vi "Test GUI.vi"() -> ()   [LabVIEW 2018]
doc: "Acoustic Test for EOL"
uses:
  Types/EnumType.ctl
  <vilib>/Utility/miscctls.llb/LVRowAndColumnTypeDef.ctl
  <vilib>/Utility/miscctls.llb/LVRowAndColumnUnsignedTypeDef.ctl
  <vilib>/Utility/error.llb/DialogType.ctl
  Supports/Global 1.vi
panel:
  out "SN":u16
  in  "ZEBRA PRINT ME74":bool
  in  "Reset Conter 2":bool
  out "TARGET COUNTER":dbl
  in  "PLAN TARGET":dbl
  out "CounterFull 2":bool
  out "Buffer 2":u16
  out "Buffer":u16
  out "MIC 2":cluster{dbl[], dbl[]}[](graph)
  out "Test Data":string[][](table)
  out "MIC 1":cluster{dbl[], dbl[]}[](graph)
  in  "Change Model":bool
  in  "Alarm":u16
  out "Alarm Display":string
  out "MCError":bool
  out "Auto Running":bool
  out "CYCLE\nTIME":u16
  out "ME79Model":bool
  in  "Reset Conter":bool
  out "NG":dbl
  out "OK":dbl
  in  "BOX TARGET":dbl
  out "CounterFull":bool
  out "File Open Reference out":T1
  out "Test Error":bool
  out "Power OK":bool
  in  "Print":bool=TRUE
  out "LBL Data":T2
  in  "Cal Mic CH":bool
  out "AT Cond 2":bool
  out "AT Cond":bool
  in  "IAI Cal":bool
  in  "IAI Ret":bool
  in  "IAI Adv":bool
  out "Status":string
  in  "Calibrate":bool
  out "Connection":bool
  out "Stop":bool
  out "Start":bool
  out "Error":bool
  out "Fail":bool
  out "Pass":bool
  out "Done":bool
  out "Busy":bool
  out "Ready":bool
  in  "Channel":bool
  out "Model":bool
  in  "Start":bool
  in  "Mode":bool
  in  "Quit":bool
  out "Test Result":bool
  out "Test Running":bool
  # "MICROPHONE TEST EOL"
  # "TEST DATA"
  # "MANUAL CONTROL"
  # "BUFFER\nE180639"
  # "BUFFER\nE183362"
  # "Version 2.1 Build 20200305"
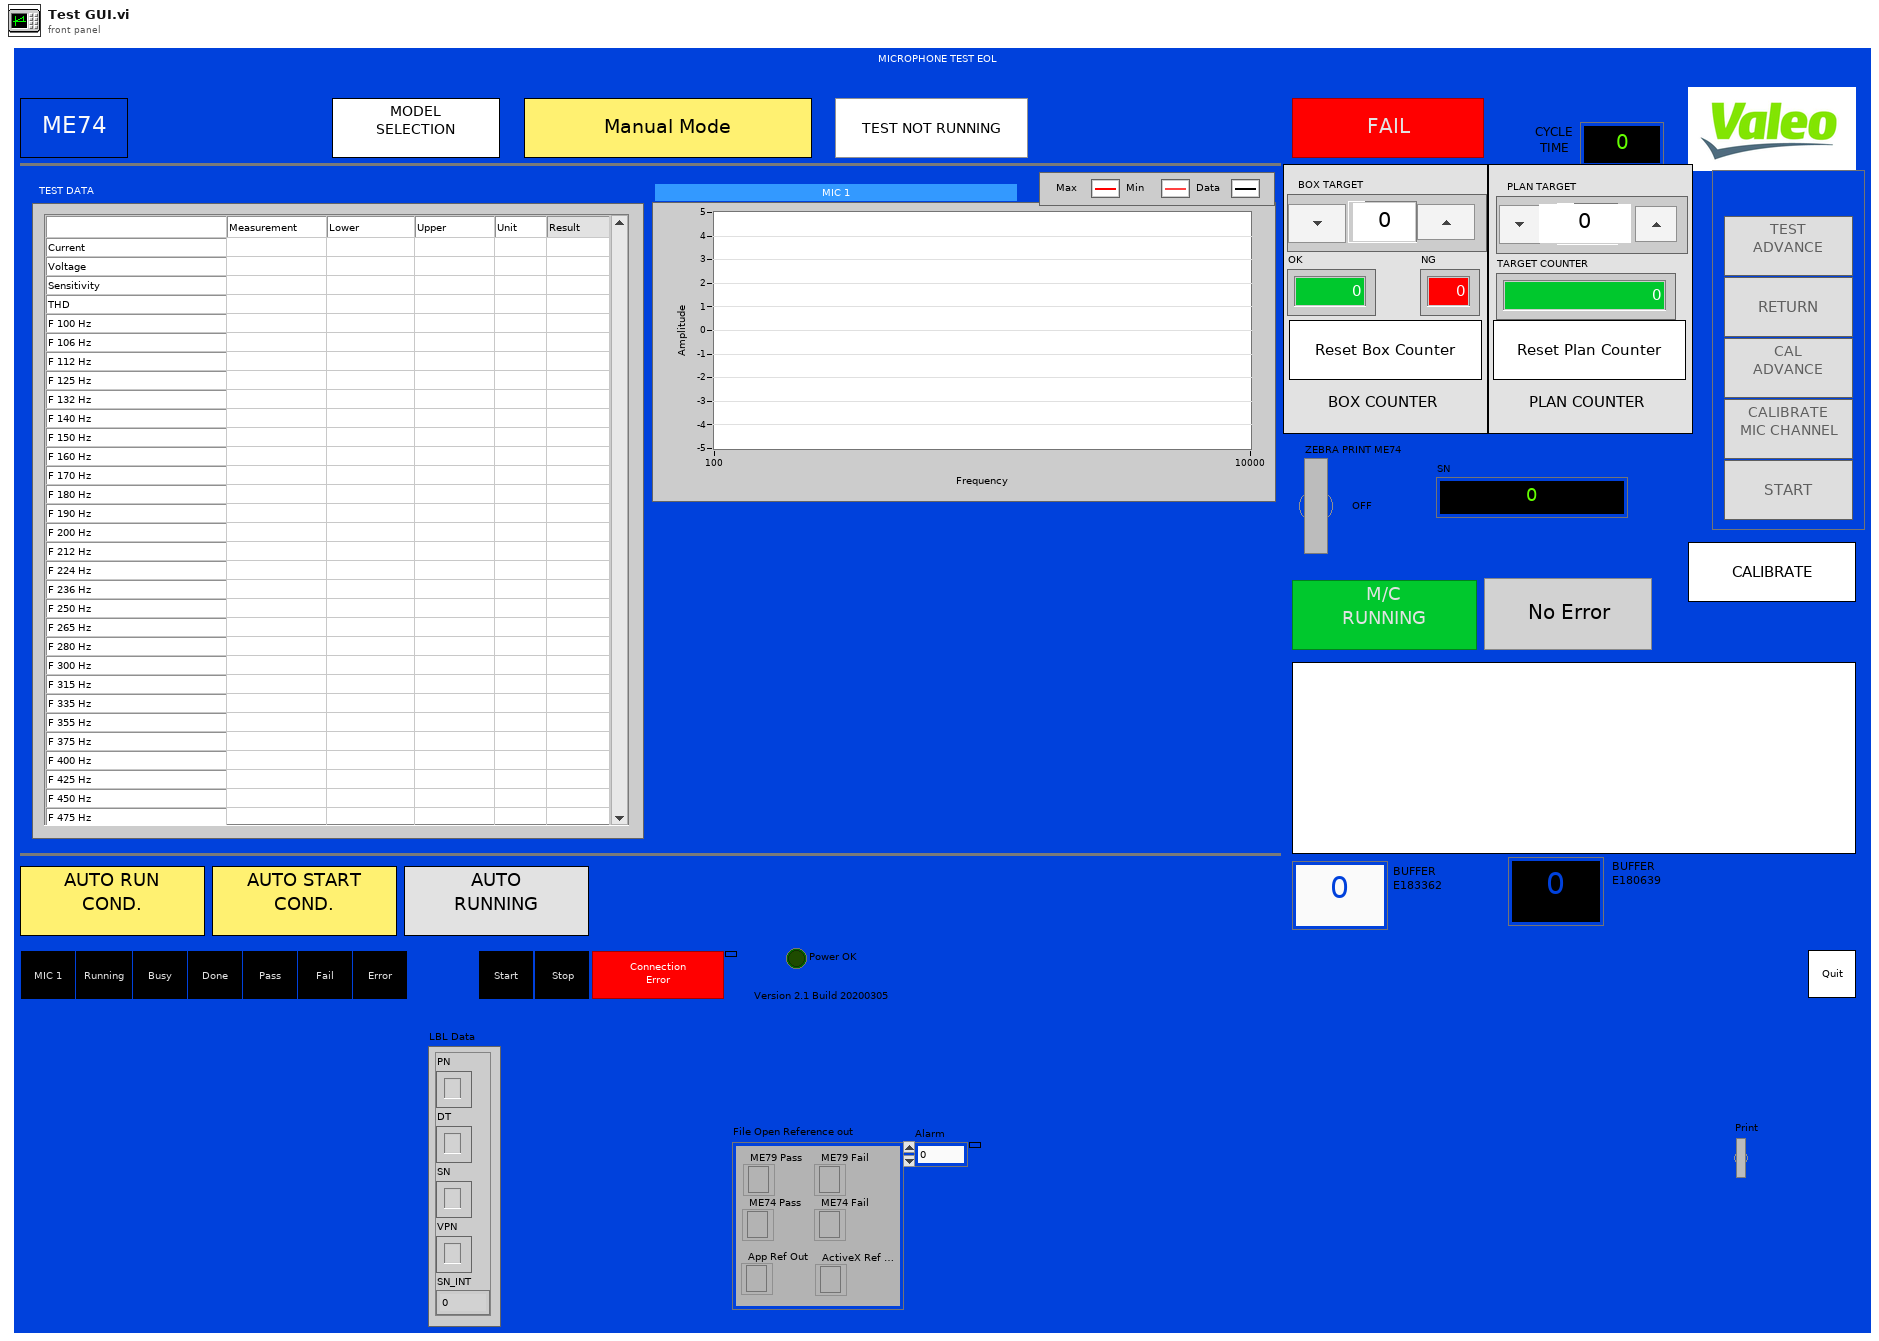
[diagram p1: front panel]
types:
  T1 = cluster{"ME79 Pass":refnum<k7>, "ME79 Fail":refnum<k7>, "ME74 Pass":refnum<k7>, "ME74 Fail":refnum<k7>, "App Ref Out":refnum<k7>, "ActiveX Ref Out":refnum<k7>}
  T2 = cluster{"PN":string, "DT":string, "SN":string, "VPN":string, "SN_INT":i32}
  T3 = typedef "EnumType.ctl" = enum16{"Initial", "Wait PLC Connect", "Ready", "Load and Init Config", "Power Supply On", "Freq Sweep 1", "Freq Sweep 2", "Power Supply Off", "Save Test Data", "Print Label", "Display Result", "Quit", "Calibration"}
  T4 = enum8{"Enabled", "Disabled", "Disabled and Grayed Out"}
  T5 = typedef "LVRowAndColumnTypeDef.ctl" = cluster{"Row":i32, "Column":i32}
  T6 = typedef "LVRowAndColumnUnsignedTypeDef.ctl" = cluster{"Row":u32, "Column":u32}
  T7 = typedef "LimitType.ctl" = cluster{"PSU":cluster{"Current Lower (mA)":dbl, "Current Upper (mA)":dbl, "Voltage Lower (V)":dbl, "Voltage Upper (V)":dbl}, "Mic":cluster{"Sensitivity (mV/Pa)":cluster{"Lower":dbl, "Upper":dbl}, "THD (%)":cluster{"Lower":dbl, "Upper":dbl}, "Freq Response":cluster{"Freq":dbl, "Upper":dbl, "Lower":dbl}[]}}
  T8 = typedef "ConfigurationType.ctl" = cluster{"PSU Setting":T9, "Sweep Settings":T10}
  T9 = typedef "SupplyConfig.ctl" = cluster{"Channel Name":string, "Source Delay (Sec)":dbl, "Measurement:Sense":i32, "voltage level":dbl, "voltage level range":dbl, "current limit":dbl, "current limit range":dbl, "resource name":refnum<k15>}
  T10 = typedef "Peiker_Stepped Sweep Settings.ctl" = cluster{"Input Settings":cluster{"IEPE min time to settle [s]":dbl, "Responce Channel Settings":cluster{"DSA response channel settings":T11, "response channel info":T12, "AI response settings":cluster{"response channel":tag, "max value [V]":dbl, "min value [V]":dbl, "terminal configuration":i32}}, "Stimulus Channel Settings":cluster{"AI stimulus settings":cluster{"stimulus channel":tag, "max value [V]":dbl, "min value [V]":dbl, "terminal configuration":i32}, "DSA stimulus channel settings":T11, "stimulus channel info":T12}}, "Output Settings":cluster{"AO source settings":cluster{"excitation channel":tag, "max value [V]":dbl, "min value [V]":dbl, "terminal configuration":i32}}}
  T11 = typedef "svc_DSA Channel Settings.ctl" = cluster{"coupling":i32, "enable IEPE excitation":bool, "IEPE current [mA]":dbl}
  T12 = typedef "svc_Channel Info.ctl" = cluster{"sensor sensitivity":dbl, "engineering units":T13, "dB reference":dbl, "custom label":string, "weighting filter":T14, "pregain":dbl}
  T13 = typedef "svc_Engineering Units Text Ring.ctl" = u16
  T14 = typedef "svc_Weighting Filter Text Ring.ctl" = u16
  T15 = cluster{"Label Data":string, "Label Data":string, "Label Data":string, "Label Data":string, "Cycle Time (ms)":i32}
  T16 = typedef "DialogType.ctl" = u16
  T17 = cluster{"frequency [Hz]":dbl[], "amplitude":dbl[]}
  T18 = cluster{string, "DT":string, "SN":string, "date/time string":string, "LINECODE":string, "NG CODE OUT":string}
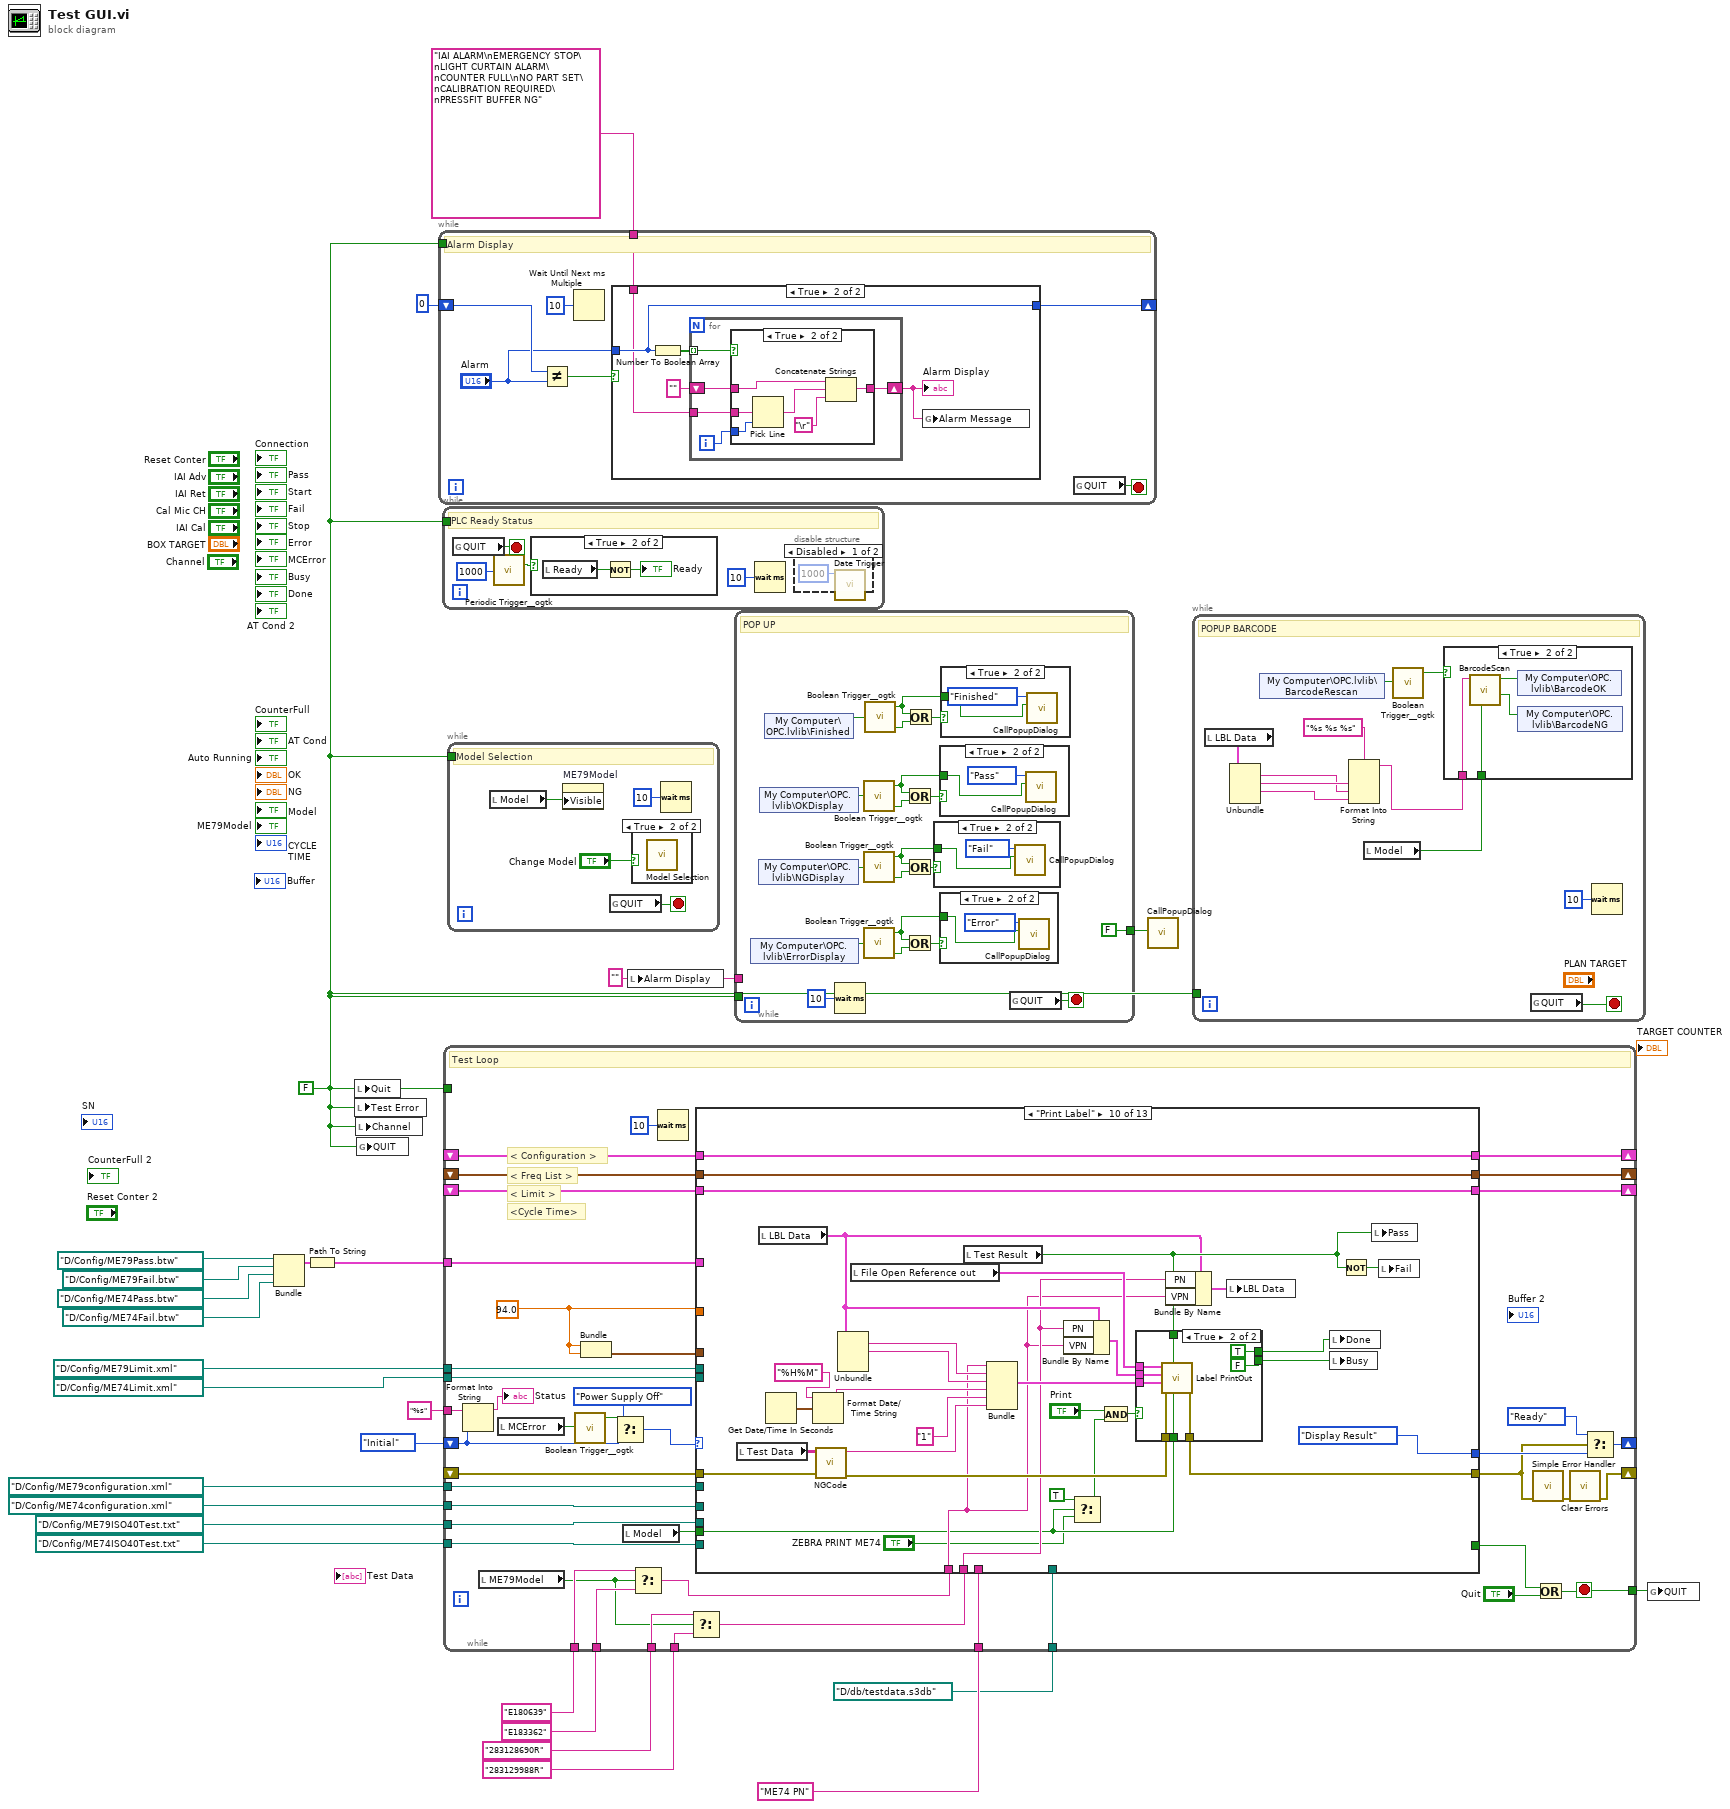
[diagram p0: block diagram]
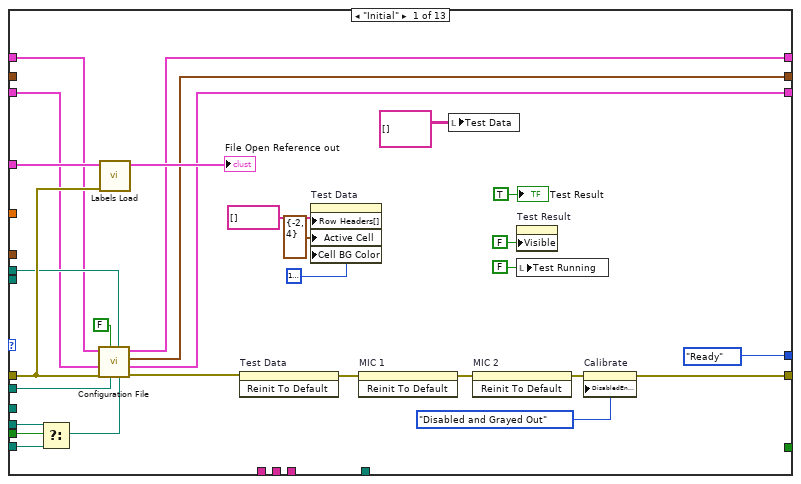
[diagram p12: hidden frame]
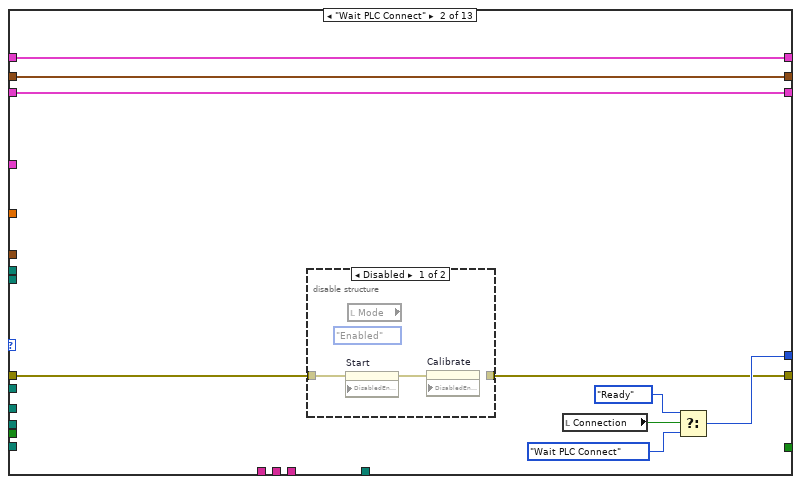
[diagram p13: hidden frame]
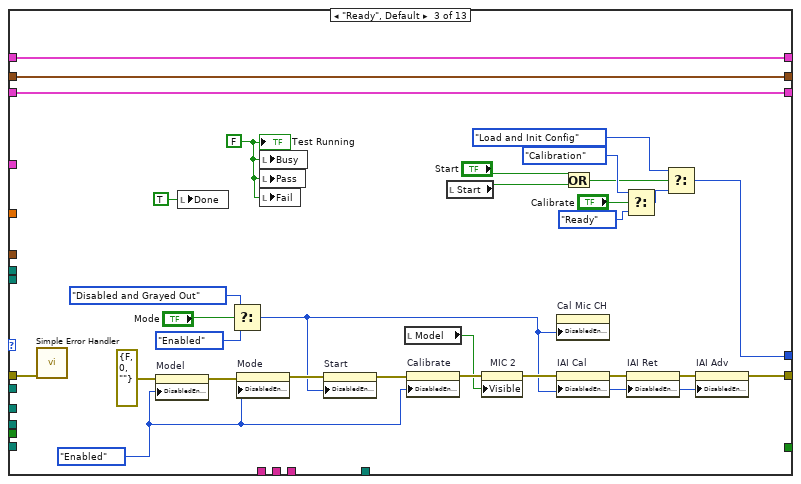
[diagram p15: hidden frame]
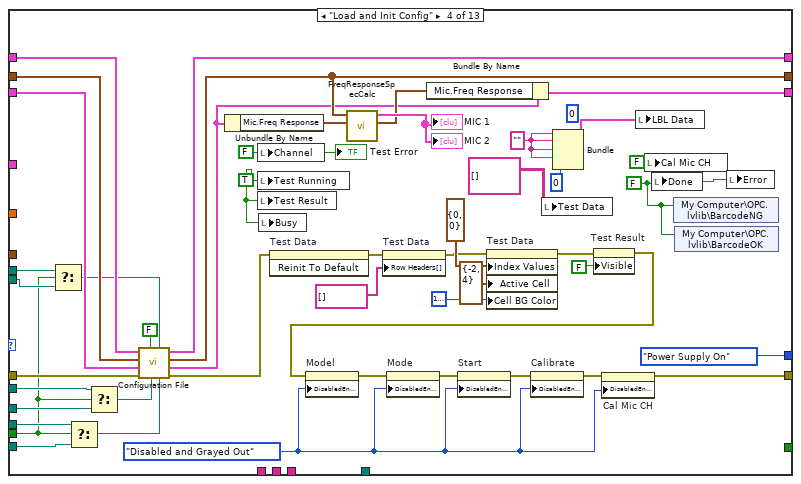
[diagram p16: hidden frame]
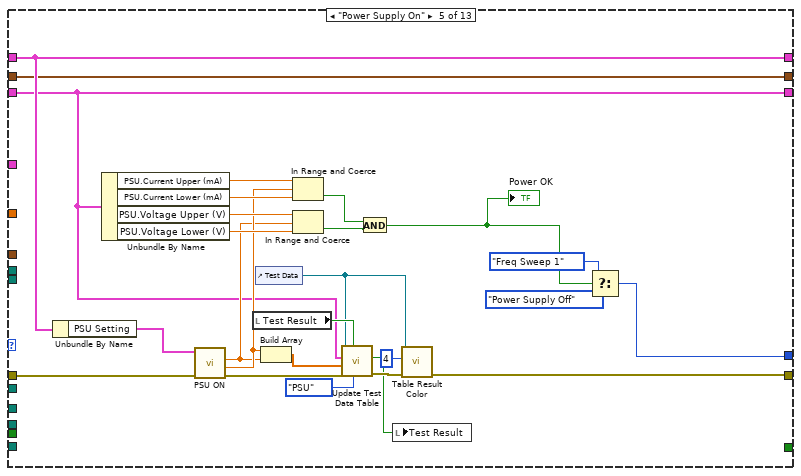
[diagram p17: hidden frame]
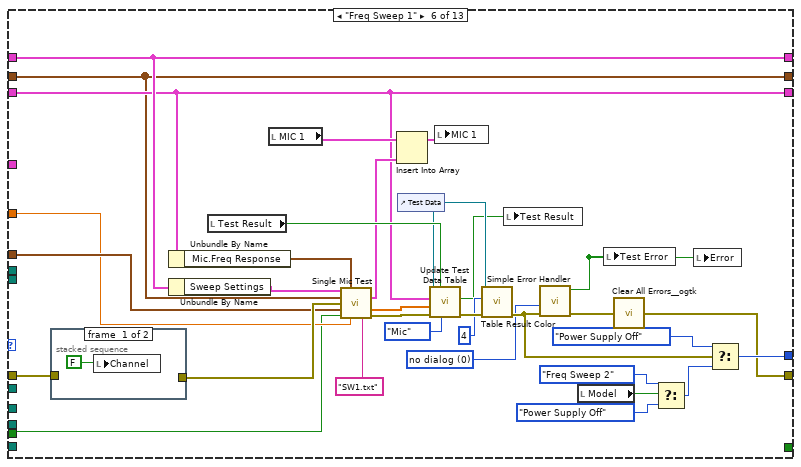
[diagram p18: hidden frame]
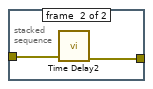
[diagram p19: hidden frame]
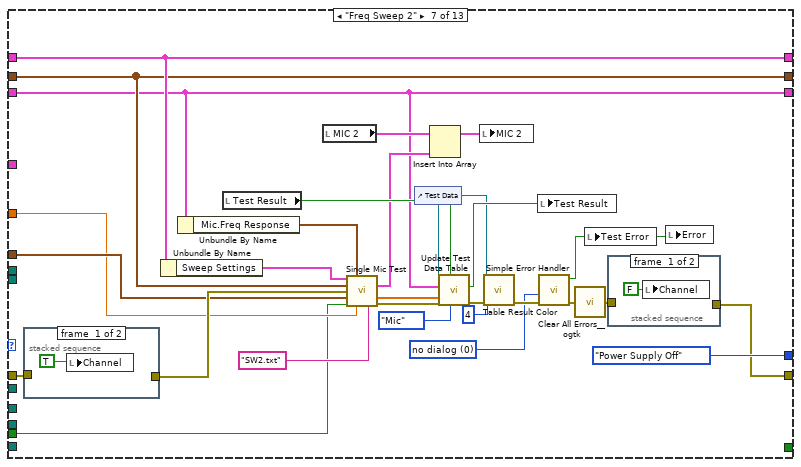
[diagram p20: hidden frame]
diagram:
  w2 = ""
  w1 = FALSE ("Quit")
  n1 = Bundle(path "D:/Config/ME79Pass.btw", path "D:/Config/ME79Fail.btw", path "D:/Config/ME74Pass.btw", path "D:/Config/ME74Fail.btw") -> (w23:cluster{path, path, path, path})  [unwired: 1 in]
  n2 = Path To String(path=w23) -> (string=w24:cluster{string, string, string, string})
  n3 = local write "Quit"(w1) -> ()
  n4 = local write "Test Error"(w1) -> ()
  n5 = local write "Channel"(w1) -> ()
  n6 = global write "Global 1.vi" "QUIT"(w1) -> ()
  n7 = while {
    shift-right: [w30] -> _
    shift-left: u16 0 -> [w32]
    tunnel: w1 -> [_]
    tunnel: "IAI ALARM\nEMERGENCY STOP\nLIGHT CURTAIN ALARM\nCOUNTER FULL\nNO PART SET\nCALIBRATION REQUIRED\nPRESSFIT BUFFER NG" -> [w28]
    stop <- w27 stop-if-true
    # "Alarm Display"
    n8 = Not Equal?(x=w32, y="Alarm") -> (x != y?=w31:bool)
    n9 = Wait Until Next ms Multiple(millisecond multiple=u32 10) -> ()  [unwired: 1 out]
    n10 = case shown="True" w31 {
      tunnel: [w34 w37] -> w30
      tunnel: "Alarm" -> [w34 w37]
      tunnel: w28 -> [_ w36]
      frame False {
      }
      frame True {
        n11 = Number To Boolean Array(number=w37) -> (Boolean array=w39:bool[])
        n12 = for {
          tunnel: w39 -> [w44] mode=indexing
          shift-right: [w41] -> w35
          shift-left: "" -> [w40]
          tunnel: w36 -> [w42]
          i -> [w43]
          n13 = case shown="True" w44 {
            tunnel: w43 -> [_ w51]
            tunnel: w42 -> [_ w50]
            tunnel: w40 -> [w45 w48]
            tunnel: [w45 w49] -> w41
            frame False {
            }
            frame True {
              n14 = Pick Line(multi-line string=w50, line index=w51) -> (output string=w47:string)  [unwired: 1 in]
              n15 = Concatenate Strings(w48, w47, "\r") -> (w49:string)
            }
          }
        }
        "Alarm Display" <- w35
        n16 = global write "Global 1.vi" "Alarm Message"(w35) -> ()
      }
    }
    n17 = global read "Global 1.vi" "QUIT"() -> (w27:bool)
  }
  n18 = while {
    tunnel: w1 -> [_]
    stop <- w52 stop-if-true
    # "PLC Ready Status"
    n19 = global read "Global 1.vi" "QUIT"() -> (w52:bool)
    n20 = call <userlib>:"Periodic Trigger__ogtk.vi"("time (ms)"=u32 1000 ("y")) -> ("Triggered"=w55:bool)  [unwired: 12 in, 2 out]
    n21 = case shown="True" w55 {
      frame False {
      }
      frame True {
        n22 = local read "Ready"() -> (w57:bool)
        n23 = Not(x=w57) -> (.not. x?=→"Ready":bool)
      }
    }
    n24 = Wait (ms)(milliseconds to wait=u32 10) -> ()  [unwired: 1 out]
    n25 = disable-structure shown="Disabled" {
      frame Disabled {
        n26 = call "Date Trigger.vi"("y"=u32 1000) -> ()  [unwired: 11 in]
      }
      frame Enabled {
      }
    }
  }
  n27 = while {
    shift-right: [w88] -> _
    shift-left: EnumType."Initial" ("Enum") -> [w71]
    shift-right: [w86] -> _
    shift-left: _ -> [w100]
    tunnel: path "D:/Config/ME79configuration.xml" -> [w99]
    shift-right: [w98] -> _
    shift-left: _ -> [w97]
    shift-right: [w95] -> _
    shift-left: _ -> [w96]
    tunnel: path "D:/Config/ME79ISO40Test.txt" -> [w94]
    shift-right: [w92] -> _
    shift-left: _ -> [w93]
    tunnel: path "D:/Config/ME79Limit.xml" -> [w91]
    tunnel: path "D:/db/testdata.s3db" -> [w85]
    tunnel: path "D:/Config/ME74ISO40Test.txt" -> [w83]
    tunnel: w1 -> [_]
    tunnel: "ME74 PN" -> [w80]
    tunnel: w24 -> [w77]
    tunnel: "E180639" -> [w75]
    tunnel: "E183362" -> [w74]
    tunnel: "283128690R" -> [w67]
    tunnel: "283129988R" -> [w66]
    tunnel: path "D:/Config/ME74configuration.xml" -> [w64]
    tunnel: path "D:/Config/ME74Limit.xml" -> [w63]
    tunnel: "%s" ("format string") -> [w60]
    tunnel: [w59] -> w3
    stop <- w59 stop-if-true
    w73 = 94.0 ("dB Reference")
    # "<Cycle Time>"
    # "< Limit >"
    # "< Freq List >"
    # "< Configuration >"
    # "Test Loop"
    n28 = Format Into String(format string=w60, w71) -> (resulting string=→"Status":string)  [unwired: 2 in, 1 out]
    n29 = local read "ME79Model"() -> (w62:bool)
    n30 = local read "MCError"() -> (w69:bool)
    n31 = call <userlib>:"Boolean Trigger__ogtk.vi"("Boolean Input"=w69) -> ("Rising Edge"=w68:bool)  [unwired: 1 in, 1 out]
    n32 = Bundle("dB Reference"=w73, "dB Reference"=w73) -> (w79:cluster{"dB Reference":dbl, "dB Reference":dbl})  [unwired: 1 in]
    n33 = Select(t=EnumType."Power Supply Off" ("Enum"), s=w68, f=w71) -> (s? t:f=w70:T3)
    n34 = local read "Model"() -> (w84:bool)
    n35 = Select(t=w75, s=w62, f=w74) -> (s? t:f=w76:string)
    n36 = Wait (ms)(milliseconds to wait=u32 10) -> ()  [unwired: 1 out]
    n37 = Select(t=w67, s=w62, f=w66) -> (s? t:f=w65:string)
    n38 = case shown="\"Print Label\"" w70 {
      tunnel: w100 -> [w115 w132 w169 w218 w245 w269 w301 w330 w361 w390 w424 w457 w464]
      tunnel: [w120 w131 w149 w186 w224 w249 w299 w332 w357 w404 w425 w457 w461] -> w78
      tunnel: [EnumType."Ready" ("Enum") w138 w164 EnumType."Power Supply On" ("Enum") w236 w252 EnumType."Power Supply Off" ("Enum") w322 EnumType."Print Label" ("Enum") EnumType."Display Result" ("Enum") EnumType."Ready" ("Enum") EnumType."Quit" ("Enum") EnumType."Ready" ("Enum")] -> w90
      tunnel: [_ _ _ _ _ _ _ _ _ _ _ TRUE _] -> w82
      tunnel: w99 -> [w113 _ _ w180 _ _ _ _ _ _ _ _ _]
      tunnel: [w106 w137 w172 w216 w229 w278 w310 w334 w364 w408 w429 w455 w472] -> w98
      tunnel: w97 -> [w105 w137 w172 w215 w229 w278 w310 w334 w364 w408 w429 w455 w472]
      tunnel: [w104 w136 w171 w193 w223 w255 w308 w336 w340 w407 w428 w454 w473] -> w95
      tunnel: w96 -> [_ w136 w171 w214 w223 w255 w308 w336 w340 w407 w428 w454 w473]
      tunnel: w94 -> [w111 _ _ w206 _ _ _ _ _ _ _ _ w469]
      tunnel: w93 -> [w102 w135 w170 w213 w222 w258 w289 w335 w363 w406 w427 w453 w474]
      tunnel: [w103 w135 w170 w209 w222 w258 w289 w335 w363 w406 w427 w453 w474] -> w92
      tunnel: w91 -> [w108 _ _ w178 _ _ _ _ _ _ _ _ _]
      tunnel: w85 -> [_ _ _ _ _ _ _ _ w360 _ _ _ w465]
      tunnel: w84 -> [w112 _ _ w176 _ w246 w282 _ w338 w382 _ _ w471]
      tunnel: w83 -> [w110 _ _ w205 _ _ _ _ _ _ _ _ w468]
      tunnel: w79 -> [_ _ _ _ _ w264 w295 _ _ _ _ _ _]
      tunnel: w73 -> [_ _ _ _ _ w263 w294 _ _ _ _ _ _]
      tunnel: w76 -> [_ _ _ _ _ _ _ _ w354 w384 _ _ _]
      tunnel: w80 -> [_ _ _ _ _ _ _ _ w353 _ _ _ _]
      tunnel: w77 -> [w117 _ _ _ _ _ _ _ _ _ _ _ _]
      tunnel: w65 -> [_ _ _ _ _ _ _ _ _ w385 _ _ _]
      tunnel: w64 -> [_ _ _ w181 _ _ _ _ _ _ _ _ _]
      tunnel: w63 -> [_ _ _ w177 _ _ _ _ _ _ _ _ _]
      frame "Initial" {
        n39 = Select(t=w111, s=w112, f=w110) -> (s? t:f=w109:path)
        n40 = call "Configuration File.vi"("Freq List File"=w109, "Limit File"=w108, "Configurtion File"=w113, "Mode (F-Read)"=FALSE, "Error In"=w115, "Limit"=w102, "Configuration"=w105) -> ("Error Out"=w114:errorcluster, "Limit Out"=w103:T7, "Freq List Out"=w104:cluster{"Freq":dbl, "Amp":dbl}[], "value"=w106:T8)  [unwired: 1 in]
        n41 = call "Labels Load.vi"("error in (no error)"=w115, "Labels"=w117) -> ("File Open Reference out"=→"File Open Reference out":T1)  [unwired: 8 in, 1 out]
        n42 = invoke on="Test Data" class="Tbl (strict)" method="Reinit To Default"(error in=w114) -> (error out=w128:errorcluster)  [unwired: 2 in, 2 out]
        n43 = property on="Test Data" class="Tbl (strict)"("Row Headers[]"=string[] [], "Active Cell"=T5 {"Row"=-2, "Column"=4} ("Active Cell:Active Cell"), "Cell BG Color"=u32 16777225) -> ()  [unwired: 2 in, 2 out]
        n44 = invoke on="MIC 1" class="XYGraph (strict)" method="Reinit To Default"(error in=w128) -> (error out=w127:errorcluster)  [unwired: 2 in, 2 out]
        n45 = local write "Test Data"(string[][] []) -> ()
        n46 = invoke on="MIC 2" class="XYGraph (strict)" method="Reinit To Default"(error in=w127) -> (error out=w121:errorcluster)  [unwired: 2 in, 2 out]
        n47 = property on="Test Result" class="Bool (strict)"("Visible"=FALSE) -> ()  [unwired: 2 in, 2 out]
        n48 = local write "Test Running"(FALSE ("Test Running")) -> ()
        n49 = property on="Calibrate" class="Bool"(error in=w121, "DisabledEnum"=T4."Disabled and Grayed Out" ("Disabled")) -> (error out=w120:errorcluster)  [unwired: 1 in, 1 out]
        "Test Result" <- TRUE ("Test Pass")
      }
      frame "Wait PLC Connect" {
        n50 = disable-structure shown="Disabled" {
          disable-tunnel: w132 -> [w141 w142]
          disable-tunnel: [_ w142] -> w131
          frame Disabled {
            (unwired) T4."Enabled" ("Disabled")
            n51 = property on="Start" class="Bool (strict)" props=["DisabledEnum"](error in=w141) -> (error out=w140:errorcluster)  [unwired: 2 in, 1 out]
            n52 = local read "Mode"() -> ()  [unwired: 1 out]
            n53 = property on="Calibrate" class="Bool" props=["DisabledEnum"](error in=w140) -> ()  [unwired: 2 in, 2 out]
          }
          frame Enabled {
          }
        }
        n54 = local read "Connection"() -> (w139:bool)
        n55 = Select(t=EnumType."Ready" ("Enum"), s=w139, f=EnumType."Wait PLC Connect" ("Enum")) -> (s? t:f=w138:T3)
      }
      frame "Ready", Default {
        w154 = T4."Enabled" ("Disabled")
        w146 = FALSE ("Test Running")
        n56 = call <vilib>:"Simple Error Handler.vi"("error in (no error)"=w169) -> ()  [unwired: 4 in, 5 out]
        n57 = property on="Model" class="Bool (strict)"(error in=errorcluster {"status"=FALSE, "code"=0, "source"=""} ("Error Out"), "DisabledEnum"=w154) -> (error out=w158:errorcluster)  [unwired: 1 in, 1 out]
        n58 = local write "Done"(TRUE ("Done")) -> ()
        n59 = Select(t=T4."Disabled and Grayed Out" ("Disabled"), s="Mode", f=T4."Enabled" ("Disabled")) -> (s? t:f=w145:T4)
        n60 = property on="Mode" class="Bool (strict)"(error in=w158, "DisabledEnum"=w154) -> (error out=w157:errorcluster)  [unwired: 1 in, 1 out]
        n61 = local write "Busy"(w146) -> ()
        n62 = local write "Pass"(w146) -> ()
        n63 = local write "Fail"(w146) -> ()
        n64 = property on="Start" class="Bool (strict)"(error in=w157, "DisabledEnum"=w145) -> (error out=w155:errorcluster)  [unwired: 1 in, 1 out]
        n65 = local read "Model"() -> (w143:bool)
        n66 = property on="Calibrate" class="Bool"(error in=w155, "DisabledEnum"=w154) -> (error out=w153:errorcluster)  [unwired: 1 in, 1 out]
        n67 = local read "Start"() -> (w144:bool)
        n68 = property on="MIC 2" class="XYGraph (strict)"(error in=w153, "Visible"=w143) -> (error out=w150:errorcluster)  [unwired: 1 in, 1 out]
        n69 = property on="Cal Mic CH" class="Bool (strict)"("DisabledEnum"=w145) -> ()  [unwired: 2 in, 2 out]
        n70 = property on="IAI Cal" class="Bool (strict)"(error in=w150, "DisabledEnum"=w145) -> (error out=w152:errorcluster)  [unwired: 1 in, 1 out]
        n71 = Or(x="Start", y=w144) -> (x .or. y?=w160:bool)
        n72 = Select(t=EnumType."Calibration" ("Enum"), s="Calibrate", f=EnumType."Ready" ("Enum")) -> (s? t:f=w165:T3)
        n73 = property on="IAI Ret" class="Bool (strict)"(error in=w152, "DisabledEnum"=w145) -> (error out=w151:errorcluster)  [unwired: 1 in, 1 out]
        n74 = Select(t=EnumType."Load and Init Config" ("Enum"), s=w160, f=w165) -> (s? t:f=w164:T3)
        n75 = property on="IAI Adv" class="Bool (strict)"(error in=w151, "DisabledEnum"=w145) -> (error out=w149:errorcluster)  [unwired: 1 in, 1 out]
        "Test Running" <- w146
      }
      frame "Load and Init Config" {
        w182 = "" ("Label Data")
        w174 = FALSE ("Done")
        (unwired) 0 ("Cycle Time (ms)")
        w183 = FALSE ("Channel")
        w189 = TRUE ("Test Running")
        w185 = T4."Disabled and Grayed Out" ("Disabled")
        n76 = Select(t=w178, s=w176, f=w177) -> (s? t:f=w175:path)
        n77 = Select(t=w206, s=w176, f=w205) -> (s? t:f=w204:path)
        n78 = Select(t=w180, s=w176, f=w181) -> (s? t:f=w179:path)
        n79 = call "Configuration File.vi"("Freq List File"=w204, "Limit File"=w175, "Configurtion File"=w179, "Mode (F-Read)"=FALSE, "Error In"=w218, "Limit"=w213, "Freq List In"=w214, "Configuration"=w215) -> ("Error Out"=w201:errorcluster, "Limit Out"=w192:T7, "Freq List Out"=w193:cluster{"Freq":dbl, "Amp":dbl}[], "value"=w216:T8)
        n80 = Unbundle By Name(w192) -> ("Mic.Freq Response"=w212:cluster{"Freq":dbl, "Upper":dbl, "Lower":dbl}[])
        n81 = local write "Channel"(w183) -> ()
        n82 = local write "Test Running"(w189) -> ()
        n83 = local write "Test Result"(w189) -> ()
        n84 = local write "Busy"(w189) -> ()
        n85 = invoke on="Test Data" class="Tbl (strict)" method="Reinit To Default"(error in=w201) -> (error out=w207:errorcluster)  [unwired: 2 in, 2 out]
        n86 = call "FreqResponseSpecCalc.vi"("Freq Response Spec In"=w212, "Freq List In"=w193) -> ("All Freq Spec Out"=w210:cluster{"Freq":dbl, "Upper":dbl, "Lower":dbl}[], "XY Graph"=→"MIC 1" →"MIC 2":cluster{dbl[], dbl[]}[])  [unwired: 8 in]
        n87 = property on="Test Data" class="Tbl (strict)"(error in=w207, "Row Headers[]"=string[] [] ("Row Header Strings[]")) -> (error out=w202:errorcluster)  [unwired: 1 in, 1 out]
        n88 = Bundle By Name(cluster=w192, "Mic.Freq Response"=w210) -> (w209:T7)
        n89 = property on="Test Data" class="Tbl (strict)"(error in=w202, "Index Values"=T6 {"Row"=0, "Column"=0}, "Active Cell"=T5 {"Row"=-2, "Column"=4} ("Active Cell:Active Cell"), "Cell BG Color"=u32 16777225) -> (error out=w191:errorcluster)  [unwired: 1 in, 1 out]
        n90 = local write "Test Data"(string[][] []) -> ()
        n91 = Bundle("Label Data"=w182, "Label Data"=w182, "Label Data"=w182, "Label Data"=w182, "Cycle Time (ms)"=0) -> (w184:T15)  [unwired: 1 in]
        n92 = property on="Test Result" class="Bool (strict)"(error in=w191, "Visible"=FALSE) -> (error out=w190:errorcluster)  [unwired: 1 in, 1 out]
        n93 = property on="Model" class="Bool (strict)"(error in=w190, "DisabledEnum"=w185) -> (error out=w199:errorcluster)  [unwired: 1 in, 1 out]
        n94 = property on="Mode" class="Bool (strict)"(error in=w199, "DisabledEnum"=w185) -> (error out=w198:errorcluster)  [unwired: 1 in, 1 out]
        n95 = property on="Start" class="Bool (strict)"(error in=w198, "DisabledEnum"=w185) -> (error out=w195:errorcluster)  [unwired: 1 in, 1 out]
        n96 = property on="Calibrate" class="Bool"(error in=w195, "DisabledEnum"=w185) -> (error out=w187:errorcluster)  [unwired: 1 in, 1 out]
        n97 = property on="Cal Mic CH" class="Bool (strict)"(error in=w187, "DisabledEnum"=w185) -> (error out=w186:errorcluster)  [unwired: 1 in, 1 out]
        n98 = local write "LBL Data"(w184) -> ()
        n99 = local write "Cal Mic CH"(FALSE ("IAI Cal 2")) -> ()
        n100 = local write "Done"(w174) -> ()
        n101 = shared-variable "My Computer\\OPC.lvlib\\BarcodeNG"(w174) -> ()  [unwired: 1 in, 1 out]
        n102 = shared-variable "My Computer\\OPC.lvlib\\BarcodeOK"(w174) -> ()  [unwired: 1 in, 1 out]
        n103 = local write "Error"(w174) -> ()
        "Test Error" <- w183
      }
      frame "Power Supply On" {
        n104 = Unbundle By Name(w229) -> ("PSU Setting"=w228:T9)
        n105 = Unbundle By Name(w222) -> ("PSU.Current Upper (mA)"=w244:dbl, "PSU.Current Lower (mA)"=w243:dbl, "PSU.Voltage Upper (V)"=w242:dbl, "PSU.Voltage Lower (V)"=w241:dbl)
        n106 = call "PSU ON.vi"("Error In"=w245, "PSU Setting"=w228) -> ("Error Out"=w235:errorcluster, "Current Result (mA)"=w234:dbl, "Volt Result"=w233:dbl)  [unwired: 6 in, 1 out]
        n107 = local read "Test Result"() -> (w231:bool)
        n108 = control-ref of="Test Data"() -> (w226:refnum<vi>)
        n109 = Build Array(w234, w233) -> (w232:dbl[])
        n110 = In Range and Coerce(upper limit=w244, x=w234, lower limit=w243) -> (In Range?=w240:bool)  [unwired: 1 out]
        n111 = In Range and Coerce(upper limit=w242, x=w233, lower limit=w241) -> (In Range?=w239:bool)  [unwired: 1 out]
        n112 = call "Update Test Data Table.vi"("Enum"=enum16{"PSU", "Mic"}."PSU", "Prev Result in"=w231, "Error In"=w235, "Test Data In"=w232, "Limit In"=w222, "Test Data ref in"=w226) -> ("Error Out"=w227:errorcluster, "Latest Result Out"=w221:bool)  [unwired: 4 in]
        n113 = And(x=w240, y=w239) -> (x .and. y?=w220:bool)
        "Power OK" <- w220
        n114 = local write "Test Result"(w221) -> ()
        n115 = call "Table Result Color.vi"("Error In"=w227, "Result Column"=4, "Table Ref"=w226) -> ("Error Out"=w224:errorcluster)  [unwired: 8 in]
        n116 = Select(t=EnumType."Freq Sweep 1" ("Enum"), s=w220, f=EnumType."Power Supply Off" ("Enum")) -> (s? t:f=w236:T3)
      }
      frame "Freq Sweep 1" {
        w247 = T16 0 items=["no dialog", "OK message", "continue or stop message", "OK message + warnings", "continue/stop + warnings"] ("type of dialog (OK msg:1)")
        n117 = stacked-sequence {
          tunnel: w269 -> [_ w281]
          tunnel: [_ w280] -> w268
          frame #0 {
            n118 = local write "Channel"(FALSE) -> ()
          }
          frame #1 {
            n119 = call "Time Delay2"("error in (no error)"=w281) -> ("error out"=w280:errorcluster)  [unwired: 10 in]
          }
        }
        n120 = Unbundle By Name(w258) -> ("Mic.Freq Response"=w257:cluster{"Freq":dbl, "Upper":dbl, "Lower":dbl}[])
        n121 = Unbundle By Name(w278) -> ("Sweep Settings"=w277:T10)
        n122 = local read "Test Result"() -> (w272:bool)
        n123 = local read "MIC 1"() -> (w261:cluster{dbl[], dbl[]}[])
        n124 = call "Single Mic Test.vi"("Peiker_Stepped Sweep Settings"=w277, "Freq Response Limit"=w257, "frequency list Input"=w255, "Error In"=w268, "Test Level"=w264, "Model (T-79)"=w246, "dB Reference"=w263, "String"="SW1.txt") -> ("Processed Freq Response"=w260:T17, "Test Result Out"=w273:dbl[], "Error Out"=w271:errorcluster)  [unwired: 4 in, 1 out]
        n125 = Insert Into Array(array=w261, new element=w260) -> (w259:cluster{dbl[], dbl[]}[])  [unwired: 1 in]
        n126 = control-ref of="Test Data"() -> (w266:refnum<vi>)
        n127 = call "Update Test Data Table.vi"("Enum"=enum16{"PSU", "Mic"}."Mic", "Prev Result in"=w272, "Error In"=w271, "Test Data In"=w273, "Limit In"=w258, "Test Data ref in"=w266) -> ("Error Out"=w267:errorcluster, "Latest Result Out"=w256:bool)  [unwired: 4 in]
        n128 = local write "MIC 1"(w259) -> ()
        n129 = call "Table Result Color.vi"("Error In"=w267, "Result Column"=4, "Table Ref"=w266) -> ("Error Out"=w251:errorcluster)  [unwired: 8 in]
        n130 = local write "Test Result"(w256) -> ()
        n131 = call <vilib>:"Simple Error Handler.vi"("type of dialog (OK msg:1)"=w247, "error in (no error)"=w251) -> ("error?"=w248:bool, "error out"=w250:errorcluster)  [unwired: 3 in, 3 out]
        n132 = local read "Model"() -> (w276:bool)
        n133 = local write "Test Error"(w248) -> ()
        n134 = call <userlib>:"Clear All Errors__ogtk.vi"("Error In"=w250) -> ("Error Out"=w249:errorcluster)  [unwired: 3 in]
        n135 = Select(t=EnumType."Freq Sweep 2" ("Enum"), s=w276, f=EnumType."Power Supply Off" ("Enum")) -> (s? t:f=w253:T3)
        n136 = local write "Error"(w248) -> ()
        n137 = Select(t=EnumType."Power Supply Off" ("Enum"), s=w251, f=w253) -> (s? t:f=w252:T3)
      }
      frame "Freq Sweep 2" {
        w283 = T16 0 items=["no dialog", "OK message", "continue or stop message", "OK message + warnings", "continue/stop + warnings"] ("type of dialog (OK msg:1)")
        n138 = stacked-sequence {
          tunnel: w301 -> [_ w317]
          tunnel: [_ w316] -> w300
          frame #0 {
            n139 = local write "Channel"(TRUE) -> ()
          }
          frame #1 {
            n140 = call "Time Delay"("error in (no error)"=w317) -> ("error out"=w316:errorcluster)  [unwired: 10 in]
          }
        }
        n141 = Unbundle By Name(w310) -> ("Sweep Settings"=w309:T10)
        n142 = Unbundle By Name(w289) -> ("Mic.Freq Response"=w288:cluster{"Freq":dbl, "Upper":dbl, "Lower":dbl}[])
        n143 = local read "Test Result"() -> (w303:bool)
        n144 = local read "MIC 2"() -> (w292:cluster{dbl[], dbl[]}[])
        n145 = call "Single Mic Test.vi"("Peiker_Stepped Sweep Settings"=w309, "Freq Response Limit"=w288, "frequency list Input"=w308, "Error In"=w300, "Test Level"=w295, "Model (T-79)"=w282, "dB Reference"=w294, "String"="SW2.txt") -> ("Processed Freq Response"=w291:T17, "Test Result Out"=w304:dbl[], "Error Out"=w305:errorcluster)  [unwired: 4 in, 1 out]
        n146 = control-ref of="Test Data"() -> (w298:refnum<vi>)
        n147 = Insert Into Array(array=w292, new element=w291) -> (w290:cluster{dbl[], dbl[]}[])  [unwired: 1 in]
        n148 = call "Update Test Data Table.vi"("Enum"=enum16{"PSU", "Mic"}."Mic", "Prev Result in"=w303, "Error In"=w305, "Test Data In"=w304, "Limit In"=w289, "Test Data ref in"=w298) -> ("Error Out"=w296:errorcluster, "Latest Result Out"=w302:bool)  [unwired: 4 in]
        n149 = local write "MIC 2"(w290) -> ()
        n150 = call "Table Result Color.vi"("Error In"=w296, "Result Column"=4, "Table Ref"=w298) -> ("Error Out"=w287:errorcluster)  [unwired: 8 in]
        n151 = local write "Test Result"(w302) -> ()
        n152 = call <vilib>:"Simple Error Handler.vi"("type of dialog (OK msg:1)"=w283, "error in (no error)"=w287) -> ("error?"=w284:bool, "error out"=w286:errorcluster)  [unwired: 3 in, 3 out]
        n153 = call <userlib>:"Clear All Errors__ogtk.vi"("Error In"=w286) -> ("Error Out"=w285:errorcluster)  [unwired: 3 in]
        n154 = local write "Test Error"(w284) -> ()
        n155 = stacked-sequence {
          tunnel: w285 -> [_ w314]
          tunnel: [_ w313] -> w299
          frame #0 {
            n156 = local write "Channel"(FALSE) -> ()
          }
          frame #1 {
            n157 = call "Time Delay3"("error in (no error)"=w314, "Delay Time (s)"=0.2) -> ("error out"=w313:errorcluster)  [unwired: 9 in]
          }
        }
        n158 = local write "Error"(w284) -> ()
      }
      frame "Power Supply Off" {
        n159 = Unbundle By Name(w334) -> ("PSU Setting.resource name"=w318:refnum<k15>)
        n160 = property on="Test Result" class="Bool (strict)"(error in=w330, "Visible"=TRUE) -> (error out=w329:errorcluster)  [unwired: 1 in, 1 out]
        n161 = control-ref of="Test Data"() -> (w326:refnum<vi>)
        n162 = call "Reset_Power_Supply.vi"("error in (no error)"=errorcluster {"status"=FALSE, "code"=0, "source"=""}, "resource name"=w318) -> ("error out"=w328:errorcluster)  [unwired: 9 in]
        n163 = call "Table Result Color.vi"("Error In"=w328, "Result Column"=4, "Table Ref"=w326) -> ("Error Out"=w327:errorcluster)  [unwired: 8 in]
        n164 = Merge Errors(w329, w327) -> (w332:errorcluster)
        n165 = local read "MCError"() -> (w321:bool)
        n166 = local read "Test Error"() -> (w320:bool)
        n167 = Or(x=w321, y=w320) -> (x .or. y?=w319:bool)
        n168 = Select(t=EnumType."Display Result" ("Enum"), s=w319, f=EnumType."Save Test Data" ("Enum")) -> (s? t:f=w322:T3)
      }
      frame "Save Test Data" {
        (unwired) string[] [] ("f")
        n169 = local read "Test Data"() -> (w350:string[][])
        n170 = for {
          tunnel: w340 -> [_] mode=indexing
          tunnel: ["0"] -> w337 mode=indexing
        }
        n171 = Index Array(array=w350, index (col)=0 ("disabled index (col)")) -> (element=w346:string[])  [unwired: 1 in]
        n172 = local read "Model"() -> (w355:bool)
        n173 = Index Array(array=w346) -> (element #1=w349:string, element #2=w348:string)  [unwired: 2 in]
        n174 = case shown="True" w338 {
          tunnel: "0" -> [w370 w375]
          tunnel: w349 -> [w369 w374]
          tunnel: w348 -> [w368 w373]
          tunnel: [w367 w372] -> w345
          tunnel: w337 -> [w366 w371]
          tunnel: w337 -> [w365 _]
          frame True {
            n175 = Build Array (concatenate)(w369, w368, w370, w370, w366, w370, w370, w365) -> (w367:string[])
          }
          frame False {
            n176 = Build Array (concatenate)(w374, w373, w375, w375, w371) -> (w372:string[])
          }
        }
        n177 = local read "Power OK"() -> (w347:bool)
        n178 = Select(t=w346, s=w347, f=w345) -> (s? t:f=w339:string[])
        n179 = local read "Test Result"() -> (w343:bool)
        n180 = Select(t=w354, s=w355, f=w353) -> (s? t:f=w352:string)
        n181 = call "Data Logger.vi"("PN In"=w352, "Test Result?"=w343, "Error In"=w361, "DB File"=w360, "Model (F-ME74)"=w355, "Test Data In"=w339) -> ("Error Out"=w358:errorcluster, "LBL Data"=w342:T2)  [unwired: 3 in, 1 out]
        "LBL Data" <- w342
        n182 = Not(x=w343) -> (.not. x?=w344:bool)
        n183 = local write "Pass"(w343) -> ()
        n184 = Unbundle By Name(w342) -> ("SN_INT"=w341:i32)
        n185 = local write "Fail"(w344) -> ()
        n186 = control-ref of="Test Data"() -> (w356:refnum<vi>)
        n187 = local write "SN"(w341) -> ()
        n188 = call "Log File.vi"("Error In"=w358, "Model (F-ME74)"=w355, "Test Data table"=w356) -> ("Error Out"=w357:errorcluster)  [unwired: 8 in]
      }
      frame "Print Label" {
        n189 = local read "Test Data"() -> (w388:string[][])
        n190 = local read "LBL Data"() -> (w386:T2)
        n191 = Get Date/Time In Seconds() -> (seconds since 1Jan1904=w400:timestamp)
        n192 = Format Date/Time String(time format string (%c)="%H%M", seconds (now)=w400) -> (date/time string=w398:string)  [unwired: 1 in]
        n193 = call "NGCode.vi"("error in (no error)"=w390, "Test Data"=w388) -> ("error out"=w389:errorcluster, "NG CODE OUT"=w387:string)  [unwired: 8 in]
        n194 = Unbundle(w386) -> ("DT"=w403:string, "SN"=w402:string)  [unwired: 3 out]
        n195 = local read "File Open Reference out"() -> (w401:T1)
        n196 = local read "Test Result"() -> (w393:bool)
        n197 = Bundle(w384, "DT"=w403, "SN"=w402, "date/time string"=w398, "LINECODE"="1", "NG CODE OUT"=w387) -> (w396:T18)  [unwired: 1 in]
        n198 = Bundle By Name(cluster=w386, "PN"=w385, "VPN"=w384) -> (w395:T2)
        n199 = Select(t=TRUE, s=w382, f="ZEBRA PRINT ME74") -> (s? t:f=w377:bool)
        n200 = And(x="Print", y=w377) -> (x .and. y?=w378:bool)
        n201 = case shown="True" w378 {
          tunnel: w389 -> [w411 w420]
          tunnel: [w411 w419] -> w404
          tunnel: w401 -> [_ w418]
          tunnel: w396 -> [_ w417]
          tunnel: w395 -> [_ w416]
          tunnel: w393 -> [_ w415]
          tunnel: w382 -> [_ w414]
          tunnel: [FALSE FALSE] -> w392
          tunnel: [TRUE TRUE] -> w391
          frame False {
          }
          frame True {
            n202 = call "Label PrintOut.vi"("Model (F-ME74)"=w414, "Label Print Pass/Fail (F-Fail)"=w415, "error in (no error)"=w420, "Fail Data"=w417, "Pass Data"=w416, "Labels Reference In"=w418) -> ("error out"=w419:errorcluster)  [unwired: 5 in]
          }
        }
        n203 = Bundle By Name(cluster=w386, "PN"=w385, "VPN"=w384) -> (w383:T2)
        n204 = local write "LBL Data"(w383) -> ()
        n205 = local write "Done"(w391) -> ()
        n206 = local write "Busy"(w392) -> ()
        n207 = Not(x=w393) -> (.not. x?=w394:bool)
        n208 = local write "Pass"(w393) -> ()
        n209 = local write "Fail"(w394) -> ()
      }
      frame "Display Result" {
        n210 = flat-sequence {
          tunnel: w424 -> [w450]
          tunnel: [w450] -> w423
          tunnel: [w445] -> w422
          frame #0 {
            n211 = local read "Test Error"() -> (w447:bool)
            n212 = local read "MCError"() -> (w446:bool)
            n213 = local write "Done"(TRUE) -> ()
            n214 = local write "Busy"(FALSE) -> ()
            n215 = Or(x=w446, y=w447) -> (x .or. y?=w445:bool)
          }
        }
        n216 = Wait (ms)(milliseconds to wait=u32 500) -> ()  [unwired: 1 out]
        n217 = disable-structure shown="Disabled" {
          disable-tunnel: [w432 w444] -> w425
          disable-tunnel: w423 -> [w431 w444]
          disable-tunnel: w422 -> [w430 _]
          frame Disabled {
            n218 = case shown="False" w430 {
              tunnel: [w434 w442] -> w432
              tunnel: w431 -> [w433 w443]
              frame False {
                n219 = local read "Test Result"() -> (w435:bool)
                n220 = case shown="True" w435 {
                  tunnel: w433 -> [w438 w441]
                  tunnel: [w437 w440] -> w434
                  frame False {
                    n221 = local write "Fail"(TRUE ("Pass")) -> ()
                    n222 = call "Fail Result.vi"("error in (no error)"=w438) -> ("error out"=w437:errorcluster)  [unwired: 10 in]
                  }
                  frame True {
                    n223 = local write "Pass"(TRUE ("Pass")) -> ()
                    n224 = call "Pass Result.vi"("error in (no error)"=w441) -> ("error out"=w440:errorcluster)  [unwired: 10 in]
                  }
                }
              }
              frame True {
                n225 = call "Error Result.vi"("error in (no error)"=w443) -> ("error out"=w442:errorcluster)  [unwired: 10 in]
              }
            }
          }
          frame Enabled {
          }
        }
      }
      frame "Quit" {
        n226 = local read "File Open Reference out"() -> (w451:T1)
        n227 = call "Close Labels.vi"("Labels Reference In"=w451) -> ()  [unwired: 10 in, 1 out]
      }
      frame "Calibration" {
        # "Do Speaker Calibration"
        n228 = case shown="False" w471 {
          tunnel: path "D:/Config/ME79ISO40.txt" -> [_ w483]
          tunnel: path "D:/Config/ME74ISO40.txt" -> [w481 _]
          tunnel: [w481 w483] -> w470
          tunnel: w469 -> [_ w482]
          tunnel: w468 -> [w480 _]
          tunnel: [w480 w482] -> w467
          frame False {
            # "ME74"
          }
          frame True {
            # "ME79"
          }
        }
        n229 = flat-sequence {
          tunnel: w464 -> [w478]
          tunnel: [w478] -> w463
          frame #0 {
            n230 = local write "Cal Mic CH"(TRUE ("IAI Cal 2")) -> ()
          }
        }
        n231 = Bundle(w470, w467) -> (w466:cluster{path, path})  [unwired: 1 in]
        n232 = call "Calibration GUI.vi"("error in (no error)"=w463, "Skip Ref Mic"=TRUE, "DB File"=w465, "File"=w466) -> ("error out"=w462:errorcluster)  [unwired: 7 in]
        n233 = flat-sequence {
          tunnel: w462 -> [w476]
          tunnel: [w476] -> w461
          frame #0 {
            n234 = local write "Cal Mic CH"(FALSE ("IAI Cal 2")) -> ()
          }
        }
      }
    }
    n235 = call <vilib>:"Simple Error Handler.vi"("error in (no error)"=w78) -> ("error out"=w87:errorcluster)  [unwired: 4 in, 4 out]
    n236 = Or(x=w82, y="Quit") -> (x .or. y?=w59:bool)
    n237 = call <vilib>:"Clear Errors.vi"("error in (no error)"=w87) -> ("error out"=w86:errorcluster)  [unwired: 5 in, 1 out]
    n238 = Select(t=EnumType."Ready" ("Enum"), s=w78, f=w90) -> (s? t:f=w88:T3)
  }
  n239 = while {
    tunnel: w1 -> [_]
    stop <- w484 stop-if-true
    # "Model Selection"
    n240 = local read "Model"() -> (w486:bool)
    n241 = property on="ME79Model" class="Bool (strict)"("Visible"=w486) -> ()  [unwired: 2 in, 2 out]
    n242 = global read "Global 1.vi" "QUIT"() -> (w484:bool)
    n243 = case shown="True" "Change Model" {
      frame False {
      }
      frame True {
        n244 = call "Model Selection.vi"() -> ()  [unwired: 12 in]
      }
    }
    n245 = Wait (ms)(milliseconds to wait=u32 10) -> ()  [unwired: 1 out]
  }
  n246 = local write "Alarm Display"(w2) -> ()
  n247 = while {
    tunnel: w1 -> [_]
    tunnel: [FALSE ("Open/Close")] -> w16
    tunnel: w2 -> [_]
    stop <- w492 stop-if-true
    # "POP UP"
    n248 = shared-variable "My Computer\\OPC.lvlib\\ErrorDisplay"() -> (w494:bool)  [unwired: 1 in, 1 out]
    n249 = shared-variable "My Computer\\OPC.lvlib\\NGDisplay"() -> (w499:bool)  [unwired: 1 in, 1 out]
    n250 = shared-variable "My Computer\\OPC.lvlib\\OKDisplay"() -> (w506:bool)  [unwired: 1 in, 1 out]
    n251 = shared-variable "My Computer\\OPC.lvlib\\Finished"() -> (w488:bool)  [unwired: 1 in, 1 out]
    n252 = Wait (ms)(milliseconds to wait=u32 10) -> ()  [unwired: 1 out]
    n253 = call <userlib>:"Boolean Trigger__ogtk.vi"("Boolean Input"=w506) -> ("Rising Edge"=w505:bool, "Falling Edge"=w503:bool)  [unwired: 1 in]
    n254 = call <userlib>:"Boolean Trigger__ogtk.vi"("Boolean Input"=w499) -> ("Rising Edge"=w500:bool, "Falling Edge"=w502:bool)  [unwired: 1 in]
    n255 = call <userlib>:"Boolean Trigger__ogtk.vi"("Boolean Input"=w494) -> ("Rising Edge"=w495:bool, "Falling Edge"=w497:bool)  [unwired: 1 in]
    n256 = call <userlib>:"Boolean Trigger__ogtk.vi"("Boolean Input"=w488) -> ("Rising Edge"=w489:bool, "Falling Edge"=w491:bool)  [unwired: 1 in]
    n257 = Or(x=w505, y=w503) -> (x .or. y?=w504:bool)
    n258 = Or(x=w500, y=w502) -> (x .or. y?=w501:bool)
    n259 = Or(x=w495, y=w497) -> (x .or. y?=w496:bool)
    n260 = Or(x=w489, y=w491) -> (x .or. y?=w490:bool)
    n261 = case shown="True" w501 {
      tunnel: w500 -> [_ w512]
      frame False {
      }
      frame True {
        n262 = call "CallPopupDialog.vi"("Open/Close"=w512, "Enum"=enum16{"Finished", "Pass", "Fail", "Error"}."Fail") -> ()  [unwired: 10 in]
      }
    }
    n263 = case shown="True" w504 {
      tunnel: w505 -> [_ w514]
      frame False {
      }
      frame True {
        n264 = call "CallPopupDialog.vi"("Open/Close"=w514, "Enum"=enum16{"Finished", "Pass", "Fail", "Error"}."Pass") -> ()  [unwired: 10 in]
      }
    }
    n265 = case shown="True" w496 {
      tunnel: w495 -> [_ w509]
      frame False {
      }
      frame True {
        n266 = call "CallPopupDialog.vi"("Open/Close"=w509, "Enum"=enum16{"Finished", "Pass", "Fail", "Error"}."Error") -> ()  [unwired: 10 in]
      }
    }
    n267 = case shown="True" w490 {
      tunnel: w489 -> [_ w508]
      frame False {
      }
      frame True {
        n268 = call "CallPopupDialog.vi"("Open/Close"=w508, "Enum"=enum16{"Finished", "Pass", "Fail", "Error"}."Finished") -> ()  [unwired: 10 in]
      }
    }
    n269 = global read "Global 1.vi" "QUIT"() -> (w492:bool)
  }
  n270 = call "CallPopupDialog.vi"("Open/Close"=w16) -> ()  [unwired: 11 in]
  n271 = while {
    tunnel: w1 -> [_]
    stop <- w518 stop-if-true
    # "POPUP BARCODE"
    n272 = local read "LBL Data"() -> (w522:T2)
    n273 = Unbundle(w522) -> ("DT"=w520:string, "SN"=w521:string, "VPN"=w519:string)  [unwired: 2 out]
    n274 = shared-variable "My Computer\\OPC.lvlib\\BarcodeRescan"() -> (w525:bool)  [unwired: 1 in, 1 out]
    n275 = Format Into String(format string="%s %s %s", w521, w520, w519) -> (resulting string=w516:string)  [unwired: 2 in, 1 out]
    n276 = local read "Model"() -> (w515:bool)
    n277 = call <userlib>:"Boolean Trigger__ogtk.vi"("Boolean Input"=w525) -> ("Rising Edge"=w524:bool)  [unwired: 1 in, 1 out]
    n278 = case shown="True" w524 {
      tunnel: w516 -> [_ w529]
      tunnel: w515 -> [_ w526]
      frame False {
      }
      frame True {
        n279 = call "BarcodeScan.vi"("Model ME79? (T-ME79)"=w526, "Barcode In"=w529) -> ("NG"=w527:bool, "OK"=w528:bool)  [unwired: 8 in]
        n280 = shared-variable "My Computer\\OPC.lvlib\\BarcodeOK"(w528) -> ()  [unwired: 1 in, 1 out]
        n281 = shared-variable "My Computer\\OPC.lvlib\\BarcodeNG"(w527) -> ()  [unwired: 1 in, 1 out]
      }
    }
    n282 = global read "Global 1.vi" "QUIT"() -> (w518:bool)
    n283 = Wait (ms)(milliseconds to wait=u32 10) -> ()  [unwired: 1 out]
  }
  n284 = global write "Global 1.vi" "QUIT"(w3) -> ()
